vi "太阳能控制器断电保存全局.vi"() -> ()   [LabVIEW 2016, in "环境动力监测库.lvlib"]
panel:
  in  "MPPT24低压告警点":dbl
  in  "MPPT12低压告警点":dbl
  in  "MPPT-24 Serial":refnum<visa-resource-name>
  in  "MPPT-12 Serial":refnum<visa-resource-name>
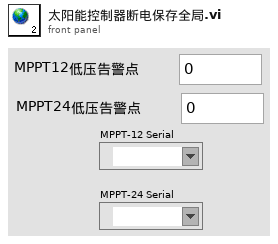
[diagram p1: front panel]
diagram:
